vi "Exit.vi"(8 "error in (no error)":errorcluster, 11 "Old State":refnum<class "UC_Idle.lvclass">) -> (0 "error out":errorcluster, 3 "New State":refnum<class "UC_Idle.lvclass">)   [LabVIEW 2025, in "User_Console.lvlib" / "UC_Idle.lvclass"]
doc: "This is an abstract method. Override this method to define the behavior when you leave the state."
uses:
  UC_Idle.lvclass
  UC_Idle.lvclass/UC_Idle.ctl
  User_Console/User_Console.lvclass
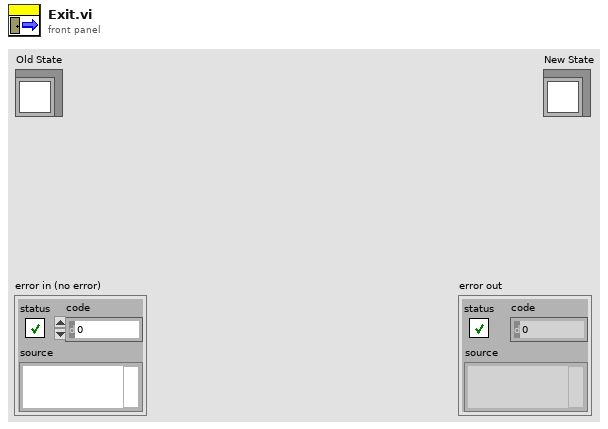
[diagram p1: front panel]
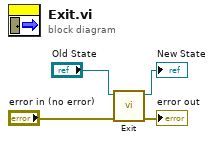
[diagram p0: block diagram]
diagram:
  n1 = call-parent "Exit.vi"("error in (no error)"="error in (no error)", "Old State"="Old State") -> ("error out"=→"error out":errorcluster, "New State"=→"New State":refnum<class "UC_Idle.lvclass">)  [unwired: 8 in]
